vi "Set Averaging Mode.vi"(9 "Averaging":i16(slide) scale=0.0..1.0, 11 "GPIB addess":string="17") -> ()   [LabVIEW 2015, in "HP4192A IA.lvclass"]
uses:
  HP4192A IA.lvclass
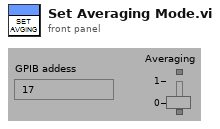
[diagram p1: front panel]
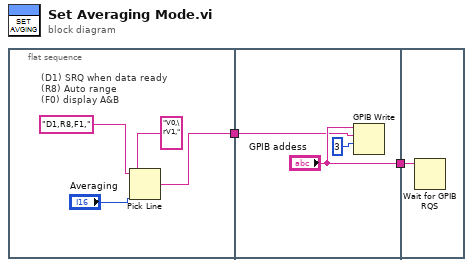
[diagram p0: block diagram]
diagram:
  n1 = flat-sequence {
    tunnel: [w3] -> w1
    tunnel: ["GPIB addess"] -> w2
    tunnel: w1 -> [w7]
    tunnel: w2 -> [w10]
    frame #0 {
      # "(D1) SRQ when data ready\n(R8) Auto range\n(F0) display A&B"
      n2 = Pick Line(string ("")="D1,R8,F1,", multi-line string="V0,\rV1,", line index="Averaging") -> (output string=w3:string)
    }
    frame #1 {
      n3 = GPIB Write(0:"GPIB addess", 1:w7, 2:3) -> ()  [unwired: 2 in, 2 out]
    }
    frame #2 {
      n4 = Wait for GPIB RQS(4:w10) -> ()  [unwired: 2 in, 2 out]
    }
  }
